vi "check x mirror speed.vi"() -> (3 "mirror speed valid":bool)   [LabVIEW 2012]
uses:
  GFG/GFGnumericGet.vi
  GFG/GFGbooleanGet.vi
  GFG/GFGfpRefGet.vi
  GFG/GFG library.lvlib
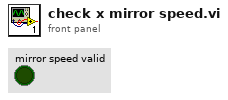
[diagram p1: front panel]
types:
  T1 = cluster{"Boolean":bool, "Numeric":dbl, "Numeric":dbl}
  T2 = cluster{"Boolean":bool, "Numeric":bool, "Numeric":bool}
  T3 = enum8{"Enabled", "Disabled", "Disabled and Grayed Out"}
  T4 = cluster{"WaveformChartRef":refnum<vi>, "DigitalRef":refnum<vi>, "ArrayRef":refnum<vi>, "TabControlRef":refnum<vi>, "EnumRef":refnum<vi>, "RingRef":refnum<vi>, "BooleanRef":refnum<vi>, "KnobRef":refnum<vi>, "SlideRef":refnum<vi>, "PathRef":refnum<vi>, "StringRef":refnum<vi>, "ComboBox":refnum<vi>, "WaveformGraphRef":refnum<vi>}
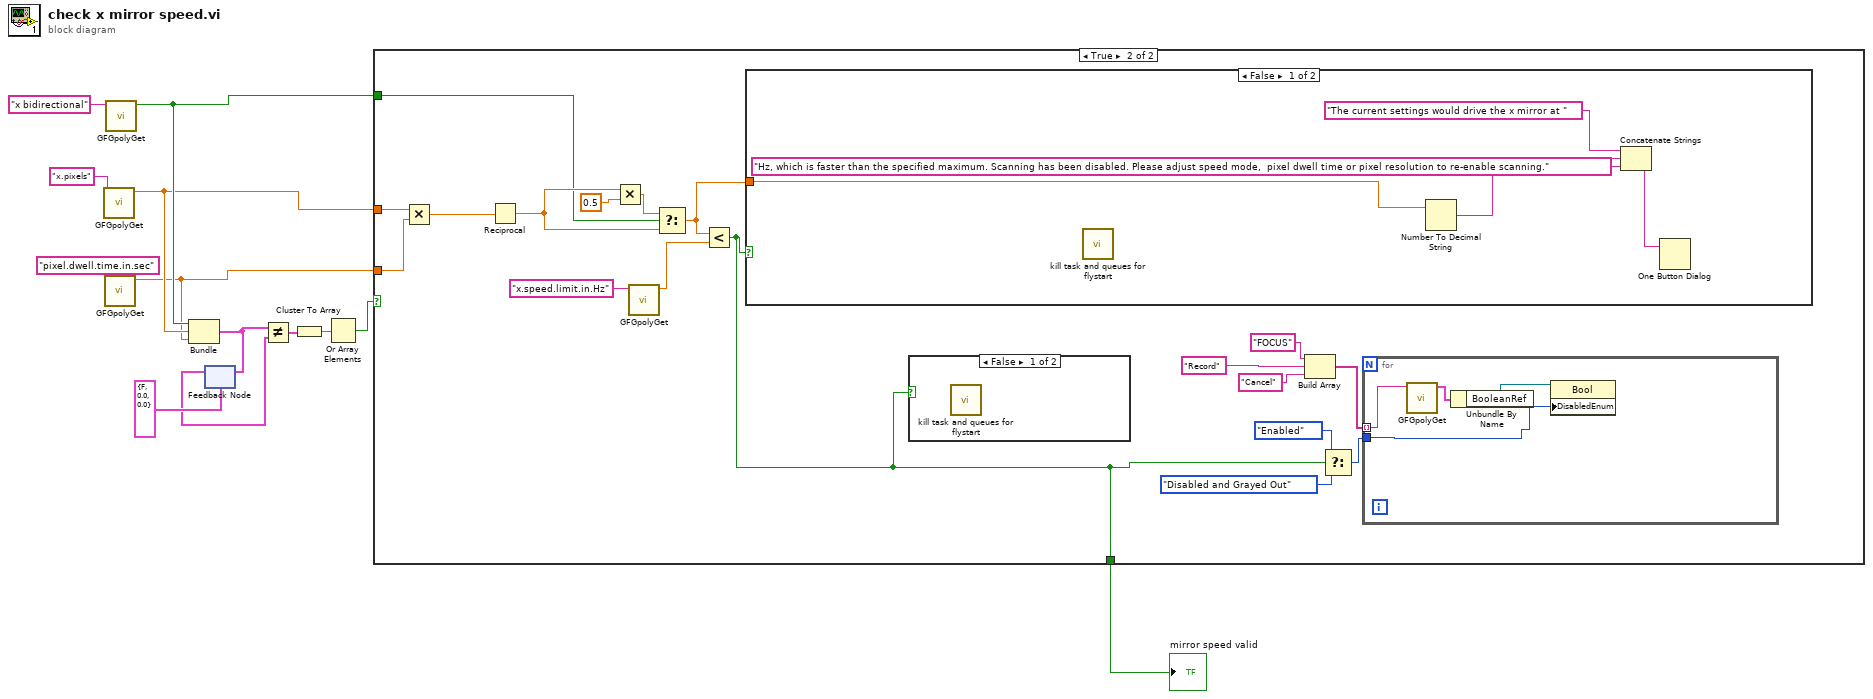
[diagram p0: block diagram]
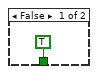
[diagram p2: hidden frame]
diagram:
  n1 = call-poly "GFGpolyGet.vi"("Variable Name in"="x.pixels") -> ("Numeric"=w9:dbl)  [unwired: 9 in, 1 out]
  n2 = call-poly "GFGpolyGet.vi"("Variable Name in"="pixel.dwell.time.in.sec") -> ("Numeric"=w8:dbl)  [unwired: 9 in, 1 out]
  n3 = call-poly "GFGpolyGet.vi"("Variable Name in"="x bidirectional") -> ("Boolean"=w10:bool)  [unwired: 10 in]
  n4 = Bundle("Boolean"=w10, "Numeric"=w9, "Numeric"=w8) -> (w6:T1)  [unwired: 1 in]
  n5 = feedback #1(T1 {"Boolean"=FALSE, "Numeric"=0.0, "Numeric"=0.0}) -> (w5:T1)
  n6 = feedback-in #1(w6) -> ()
  n7 = Not Equal?(x=w6, y=w5) -> (x != y?=w4:T2)
  n8 = Cluster To Array(cluster=w4) -> (array=w2:bool[])
  n9 = Or Array Elements(Boolean array=w2) -> (logical OR=w3:bool)
  n10 = case shown="True" w3 {
    tunnel: w10 -> [_ w27]
    tunnel: w9 -> [_ w25]
    tunnel: w8 -> [_ w24]
    tunnel: [TRUE w15] -> w1
    frame False {
    }
    frame True {
      n11 = Multiply(x=w25, y=w24) -> (x*y=w26:dbl)
      n12 = Reciprocal(x=w26) -> (1/x=w28:dbl)
      n13 = Multiply(x=w28, y=0.5) -> (x*y=w29:dbl)
      n14 = call-poly "GFGpolyGet.vi"("Variable Name in"="x.speed.limit.in.Hz") -> ("Numeric"=w32:dbl)  [unwired: 9 in, 1 out]
      n15 = Select(t=w29, s=w27, f=w28) -> (s? t:f=w17:dbl)
      n16 = Less?(x=w17, y=w32) -> (x < y?=w15:bool)
      n17 = case shown="False" w15 {
        tunnel: w17 -> [w41 _]
        frame False {
          n18 = call "kill task and queues for flystart.vi"() -> ()  [unwired: 12 in]
          n19 = Number To Decimal String(number=w41) -> (decimal integer string=w39:string)  [unwired: 1 in]
          n20 = Concatenate Strings("The current settings would drive the x mirror at " ("message"), w39, "Hz, which is faster than the specified maximum. Scanning has been disabled. Please adjust speed mode,  pixel dwell time or pixel resolution to re-enable scanning." ("string")) -> (w37:string)
          n21 = One Button Dialog(message=w37) -> ()  [unwired: 1 in, 1 out]
        }
        frame True {
        }
      }
      n22 = case shown="False" w15 {
        frame False {
          n23 = call "kill task and queues for flystart.vi"() -> ()  [unwired: 12 in]
        }
        frame True {
        }
      }
      n24 = Build Array("FOCUS" ("Variable Name in"), "Record" ("element"), "Cancel" ("element")) -> (w23:string[])
      n25 = Select(t=T3."Enabled" ("Disabled"), s=w15, f=T3."Disabled and Grayed Out" ("Disabled")) -> (s? t:f=w18:T3)
      n26 = for {
        tunnel: w23 -> [w34] mode=indexing
        tunnel: w18 -> [w33]
        n27 = call-poly "GFGpolyGet.vi"("Variable Name in"=w34) -> ("output cluster"=w36:T4)  [unwired: 9 in, 1 out]
        n28 = Unbundle By Name(w36) -> ("BooleanRef"=w35:refnum<vi>)
        n29 = property class="Bool"(reference=w35, "DisabledEnum"=w33) -> ()  [unwired: 1 in, 2 out]
      }
    }
  }
  "mirror speed valid" <- w1
